vi "密码权限设置.vi"(10 "权限输入":enum16{"一级权限", "二级权限", "三级权限", "超级权限"}(ring), 11 "权限密码":u32[](array[numeric])) -> (3 "权限输出":enum16{"一级权限", "二级权限", "三级权限", "超级权限"}(ring))   [LabVIEW 2016, in "斯坦道通用流路CODmn.lvlib"]
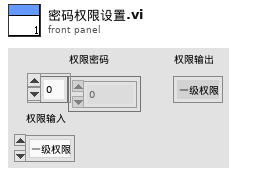
[diagram p1: front panel]
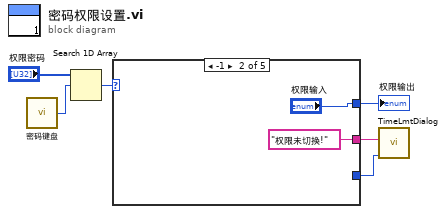
[diagram p0: block diagram]
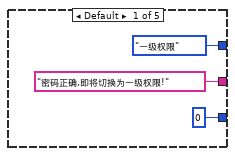
[diagram p2: hidden frame]
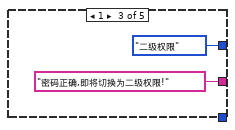
[diagram p3: hidden frame]
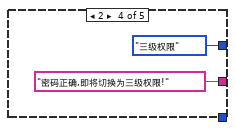
[diagram p4: hidden frame]
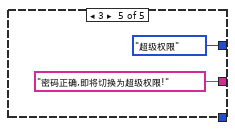
[diagram p5: hidden frame]
diagram:
  n1 = call "密码键盘.vi"() -> ("NewNumber"=w5:u32)  [unwired: 1 in]
  n2 = Search 1D Array(1D array="权限密码", element=w5) -> (index of element=w6:i32)  [unwired: 1 in]
  n3 = case shown="-1" w6 {
    tunnel: ["密码正确,即将切换为一级权限!" ("Infoin") "权限未切换!" ("Infoin") "密码正确,即将切换为二级权限!" ("Infoin") "密码正确,即将切换为三级权限!" ("Infoin") "密码正确,即将切换为超级权限!" ("Infoin")] -> w1
    tunnel: [u32 0 ("颜色盒") _ _ _ _] -> w2
    tunnel: [enum16{"一级权限", "二级权限", "三级权限", "超级权限"}."一级权限" ("权限") "权限输入" enum16{"一级权限", "二级权限", "三级权限", "超级权限"}."二级权限" ("权限") enum16{"一级权限", "二级权限", "三级权限", "超级权限"}."三级权限" ("权限") enum16{"一级权限", "二级权限", "三级权限", "超级权限"}."超级权限" ("权限")] -> w3
    frame Default {
    }
    frame -1 {
    }
    frame 1 {
    }
    frame 2 {
    }
    frame 3 {
    }
  }
  "权限输出" <- w3
  n4 = call "TimeLmtDialog.vi"("颜色盒"=w2, "Infoin"=w1) -> ()  [unwired: 10 in]
